vi "力特性 不灵敏区扭矩.vi"(8 "油压B":dbl[](array[numeric]), 9 "油压A":dbl[](array[numeric]), 10 "扭矩B":dbl[](array[numeric]), 11 "扭矩A":dbl[](array[numeric])) -> (3 "不灵敏区扭矩":dbl)   [LabVIEW 2015, in "Logging.lvlib"]
uses:
  Logging.lvlib
  <vilib>/Analysis/1siggen.llb/Ramp Pattern by Samples.vi
  <vilib>/Analysis/NI_AALBase.lvlib
  <vilib>/gmath/NI_Gmath.lvlib
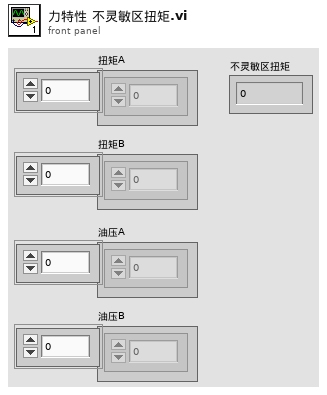
[diagram p1: front panel]
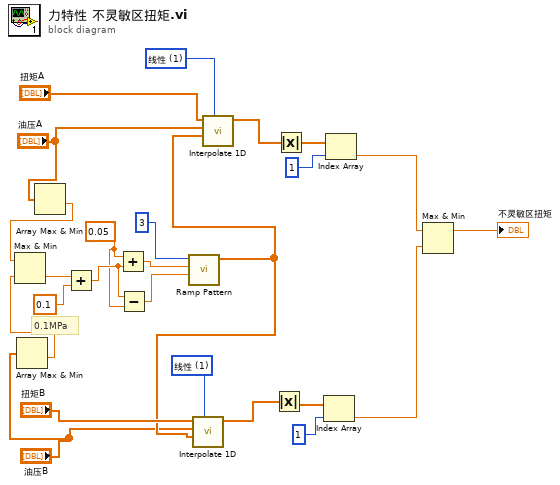
[diagram p0: block diagram]
diagram:
  w3 = 0.05 ("x")
  w19 = 1 items=["最近", "线性", "样条", "cubic Hermite", "拉格朗日"] ("method")
  w22 = 1 items=["最近", "线性", "样条", "cubic Hermite", "拉格朗日"] ("method")
  # "0.1MPa"
  n1 = Array Max & Min(array="油压B") -> (min value=w7:dbl)  [unwired: 3 out]
  n2 = Array Max & Min(array="油压A") -> (min value=w8:dbl)  [unwired: 3 out]
  n3 = Max & Min(x=w8, y=w7) -> (min(x,y)=w5:dbl)  [unwired: 1 out]
  n4 = Add(x=w5, y=0.1) -> (x+y=w4:dbl)
  n5 = Add(x=w3, y=w4) -> (x+y=w2:dbl)
  n6 = Subtract(x=w4, y=w3) -> (x-y=w1:dbl)
  n7 = call-poly <vilib>:"Ramp Pattern.vi"("start"=w1, "end"=w2, "samples"=3) -> ("Ramp Pattern"=w20:dbl[])  [unwired: 7 in, 1 out]
  n8 = call <vilib>:"Interpolate 1D.vi"("method"=w19, "xi"=w20, "X"="油压B", "Y"="扭矩B") -> ("yi"=w17:dbl[])  [unwired: 5 in, 2 out]
  n9 = call <vilib>:"Interpolate 1D.vi"("method"=w22, "xi"=w20, "X"="油压A", "Y"="扭矩A") -> ("yi"=w18:dbl[])  [unwired: 5 in, 2 out]
  n10 = Absolute Value(x=w17) -> (abs(x)=w14:dbl[])
  n11 = Absolute Value(x=w18) -> (abs(x)=w16:dbl[])
  n12 = Index Array(array=w14, index=1 ("索引")) -> (element=w11:dbl)
  n13 = Index Array(array=w16, index=1 ("索引")) -> (element=w12:dbl)
  n14 = Max & Min(x=w12, y=w11) -> (max(x,y)=→"不灵敏区扭矩":dbl)  [unwired: 1 out]
